vi "Remove Header.vi"(8 "error in (no error)":errorcluster, 10 "header":string(combo)="User-Agent", 11 "HTTP Client Advanced in":refnum<class "HTTP Client Advanced.lvclass">) -> (0 "error out":errorcluster, 3 "HTTP Client Advanced out":refnum<class "HTTP Client Advanced.lvclass">)   [LabVIEW 2021, in "HTTP Client Advanced.lvclass"]
uses:
  HTTP Client Advanced.lvclass
  HTTP Client Advanced.lvclass/HTTP Client Advanced.ctl
  <vilib>/NI/Advanced HTTP Client/Session.lvclass
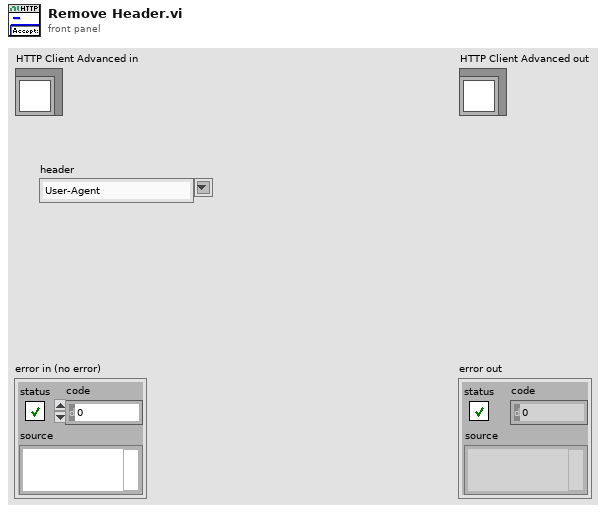
[diagram p1: front panel]
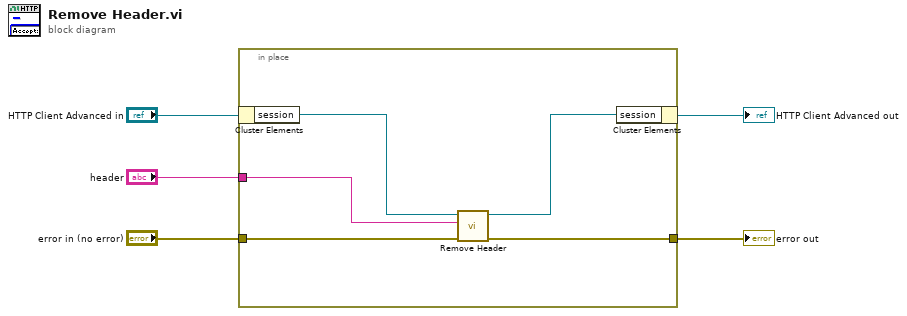
[diagram p0: block diagram]
diagram:
  n1 = in-place {
    in-place-border: "error in (no error)" -> [w10]
    in-place-border: [w9] -> w4
    in-place-border: "header" -> [w6]
    n2 = in-place-cluster #1("HTTP Client Advanced in") -> ("session"=w8:refnum<class "Session.lvclass">)
    n3 = call <vilib>:"Remove Header.vi"("error in"=w10, "header"=w6, "session in"=w8) -> ("error out"=w9:errorcluster, "session out"=w7:refnum<class "Session.lvclass">)  [unwired: 7 in]
    n4 = in-place-cluster #1("session"=w7) -> (→"HTTP Client Advanced out":refnum<class "HTTP Client Advanced.lvclass">)
  }
  "error out" <- w4
